vi "Moving_Avg.vi"(10 "Num_Avg":dbl, 11 "Numeric in":dbl) -> (3 "Numeric out":dbl)   [LabVIEW 2016, in "ArgoBotLib.lvlib"]
uses:
  ArgoBotLib.lvlib
panel:
  out "?":cluster{dbl, dbl}(graph)
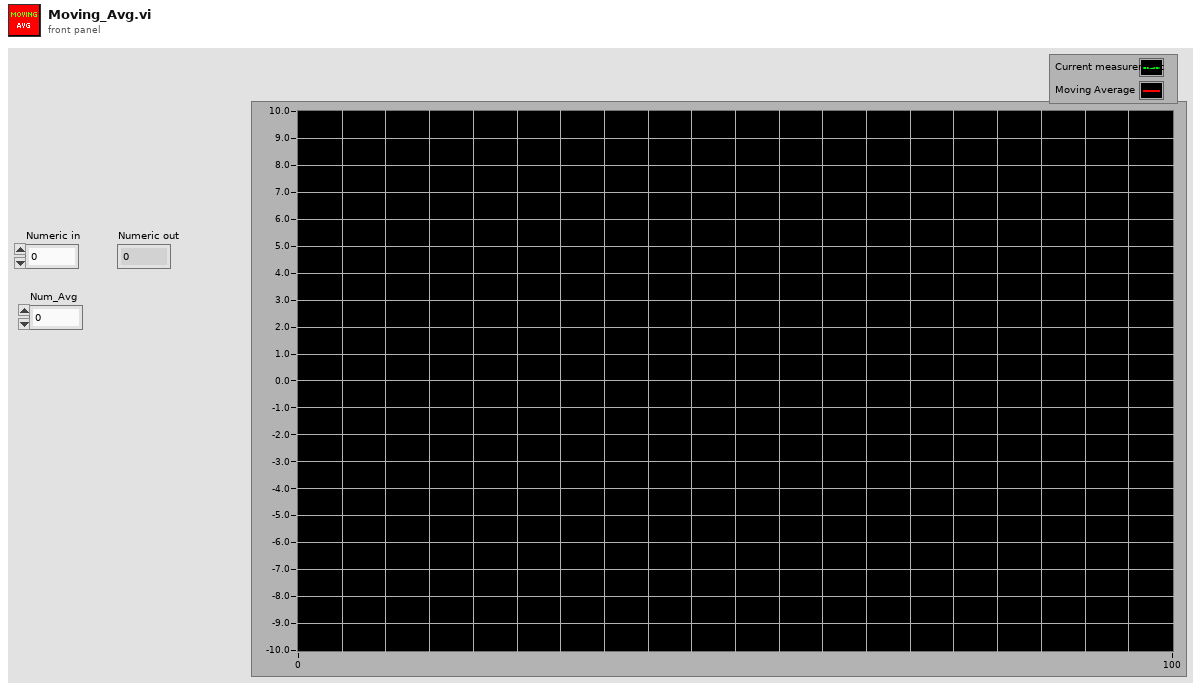
[diagram p1: front panel]
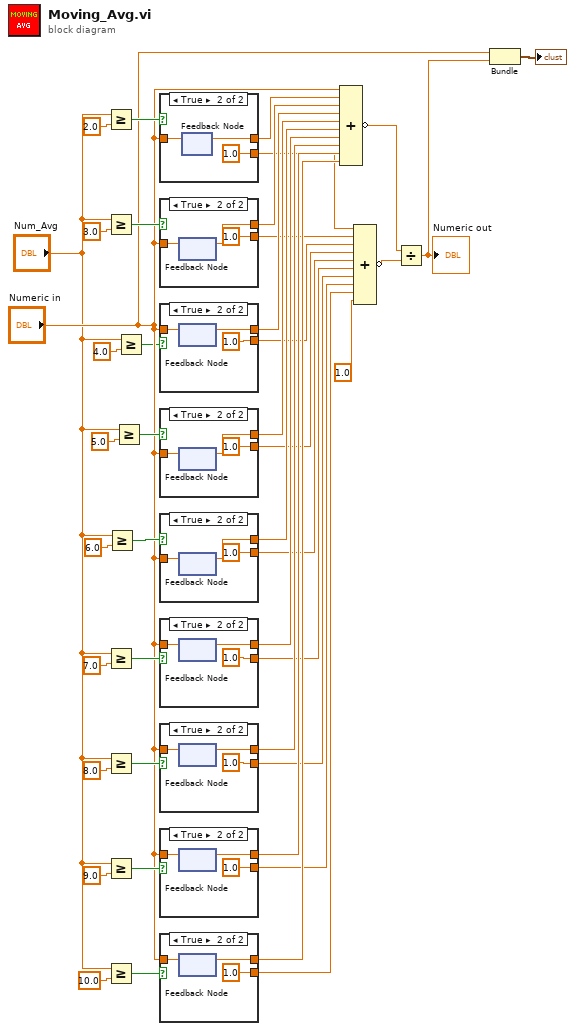
[diagram p0: block diagram]
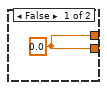
[diagram p2: hidden frame]
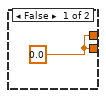
[diagram p3: hidden frame]
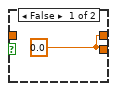
[diagram p4: hidden frame]
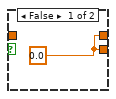
[diagram p5: hidden frame]
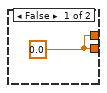
[diagram p6: hidden frame]
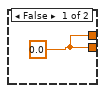
[diagram p7: hidden frame]
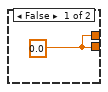
[diagram p8: hidden frame]
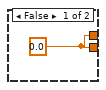
[diagram p9: hidden frame]
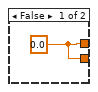
[diagram p10: hidden frame]
diagram:
  n1 = Greater Or Equal?(x="Num_Avg", y=2.0) -> (x >= y?=w42:bool)
  n2 = Greater Or Equal?(x="Num_Avg", y=3.0) -> (x >= y?=w41:bool)
  n3 = Greater Or Equal?(x="Num_Avg", y=7.0) -> (x >= y?=w38:bool)
  n4 = Greater Or Equal?(x="Num_Avg", y=8.0) -> (x >= y?=w37:bool)
  n5 = Greater Or Equal?(x="Num_Avg", y=9.0) -> (x >= y?=w36:bool)
  n6 = Greater Or Equal?(x="Num_Avg", y=10.0) -> (x >= y?=w35:bool)
  n7 = Greater Or Equal?(x="Num_Avg", y=6.0) -> (x >= y?=w39:bool)
  n8 = Greater Or Equal?(x="Num_Avg", y=5.0) -> (x >= y?=w40:bool)
  n9 = Greater Or Equal?(x="Num_Avg", y=4.0) -> (x >= y?=w2:bool)
  n10 = case shown="True" w42 {
    tunnel: "Numeric in" -> [_ w47]
    tunnel: [w44 w46] -> w26
    tunnel: [w44 1.0] -> w17
    frame False {
      w44 = 0.0
    }
    frame True {
      n11 = feedback #1() -> (w46:dbl)  [unwired: 1 in]
      n12 = feedback-in #1(w47) -> ()
    }
  }
  n13 = case shown="True" w41 {
    tunnel: "Numeric in" -> [_ w51]
    tunnel: [w48 w50] -> w25
    tunnel: [w48 1.0] -> w16
    frame False {
      w48 = 0.0
    }
    frame True {
      n14 = feedback #2() -> (w50:dbl)  [unwired: 1 in]
      n15 = feedback-in #2(w51) -> ()
    }
  }
  n16 = case shown="True" w2 {
    tunnel: "Numeric in" -> [_ w55]
    tunnel: [w52 w54] -> w24
    tunnel: [w52 1.0] -> w15
    frame False {
      w52 = 0.0
    }
    frame True {
      n17 = feedback #3() -> (w54:dbl)  [unwired: 1 in]
      n18 = feedback-in #3(w55) -> ()
    }
  }
  n19 = case shown="True" w40 {
    tunnel: "Numeric in" -> [_ w59]
    tunnel: [w56 w58] -> w23
    tunnel: [w56 1.0] -> w14
    frame False {
      w56 = 0.0
    }
    frame True {
      n20 = feedback #4() -> (w58:dbl)  [unwired: 1 in]
      n21 = feedback-in #4(w59) -> ()
    }
  }
  n22 = case shown="True" w39 {
    tunnel: "Numeric in" -> [_ w63]
    tunnel: [w60 w62] -> w22
    tunnel: [w60 1.0] -> w13
    frame False {
      w60 = 0.0
    }
    frame True {
      n23 = feedback #5() -> (w62:dbl)  [unwired: 1 in]
      n24 = feedback-in #5(w63) -> ()
    }
  }
  n25 = case shown="True" w38 {
    tunnel: "Numeric in" -> [_ w67]
    tunnel: [w64 w66] -> w21
    tunnel: [w64 1.0] -> w12
    frame False {
      w64 = 0.0
    }
    frame True {
      n26 = feedback #6() -> (w66:dbl)  [unwired: 1 in]
      n27 = feedback-in #6(w67) -> ()
    }
  }
  n28 = case shown="True" w37 {
    tunnel: "Numeric in" -> [_ w71]
    tunnel: [w68 w70] -> w20
    tunnel: [w68 1.0] -> w11
    frame False {
      w68 = 0.0
    }
    frame True {
      n29 = feedback #7() -> (w70:dbl)  [unwired: 1 in]
      n30 = feedback-in #7(w71) -> ()
    }
  }
  n31 = case shown="True" w36 {
    tunnel: "Numeric in" -> [_ w75]
    tunnel: [w72 w74] -> w19
    tunnel: [w72 1.0] -> w10
    frame False {
      w72 = 0.0
    }
    frame True {
      n32 = feedback #8() -> (w74:dbl)  [unwired: 1 in]
      n33 = feedback-in #8(w75) -> ()
    }
  }
  n34 = case shown="True" w35 {
    tunnel: "Numeric in" -> [_ w79]
    tunnel: [w76 w78] -> w18
    tunnel: [w76 1.0] -> w9
    frame False {
      w76 = 0.0
    }
    frame True {
      n35 = feedback #9() -> (w78:dbl)  [unwired: 1 in]
      n36 = feedback-in #9(w79) -> ()
    }
  }
  n37 = Compound Arithmetic op=ADD("Numeric in", w26, w25, w24, w23, w22, w21, w20, w19, w18) -> (invert w43:dbl)
  n38 = Compound Arithmetic op=ADD(w17, w16, w15, w14, w13, w12, w11, w10, w9, 1.0) -> (invert w8:dbl)
  n39 = Divide(x=w43, y=w8) -> (x/y=w6:dbl)
  "Numeric out" <- w6
  n40 = Bundle("Numeric in"="Numeric in", w6) -> (→"?":cluster{"Numeric in":dbl, dbl})  [unwired: 1 in]
